vi "test FFT sound.vi"() -> ()   [LabVIEW 2013]
uses:
  <vilib>/measure/maspectr.llb/Power Spectrum and PSD Export Mode.ctl
  <vilib>/DAQmx/read.llb/DAQmx Read (Analog Wfm 1Chan NSamp).vi
  <vilib>/Analysis/2dsp.llb/Real FFT.vi
  <vilib>/Analysis/2dsp.llb/Power Spectrum (DBL).vi
  <vilib>/DAQmx/create/channels.llb/DAQmx Create Channel (AI-Voltage-Basic).vi
  <vilib>/DAQmx/configure/timing.llb/DAQmx Timing (Sample Clock).vi
  <vilib>/DAQmx/miscellaneous.llb/DAQmx Fill In Error Info.vi
  <vilib>/express/express analysis/Spectral/Block/exnSpectralBlock spectral measurements power poly.vi
  <vilib>/express/express analysis/Spectral/Block/exnSpectralBlock spectral measurements power WFM.vi
  <vilib>/measure/maspectr.llb/FFT Power Spectrum and PSD for 1 Chan.vi
  <vilib>/measure/maspectr.llb/FFT Spectrum (Mag-Phase) for 1 Chan.vi
  <vilib>/measure/maspectr.llb/FFT Spectrum (Real-Im) for 1 Chan.vi
  <vilib>/express/express analysis/Spectral/XNode/ExpressSpectralMeasurementsBlockNode.xnode
  <vilib>/Analysis/NI_AALPro.lvlib
  <vilib>/measure/NI_MAPro.lvlib
panel:
  out "Waveform Graph":cluster{"f0":dbl, "df":dbl, "magnitude":dbl[]}(graph)
  out "element":string
  in  "index (row)":i32
  in  "spectrum units table":string[][](table)=[["FFT", "N * V", "N/2 * Vpk"], ["Power Spectrum", "V^2", "1/2 * Vrms^2"], ["Auto Power Spectrum", "V^2", "Vrms^2"], ["Amplitude and Phase Spectrum", "V", "Vrms"], ["FFT Power Spectrum", "V^2", "Vrms^2"], ["FFT Power Spectral Density", "V^2/Hz", "Vrms^2/Hz"], ["FFT Spectrum (Mag-Phase)", "V", "Vrms"], ["FFT Spectrum (Real-Imag)", "V", "Vrms"]]
  in  "stop":bool
  out "phase spectrum":dbl[](array[numeric])
  out "spectral plot":cluster{"t":dbl, "t":dbl, "magnitude":dbl[]}(graph)={"t"=0.0, "t"=1.0, "magnitude"=[]}
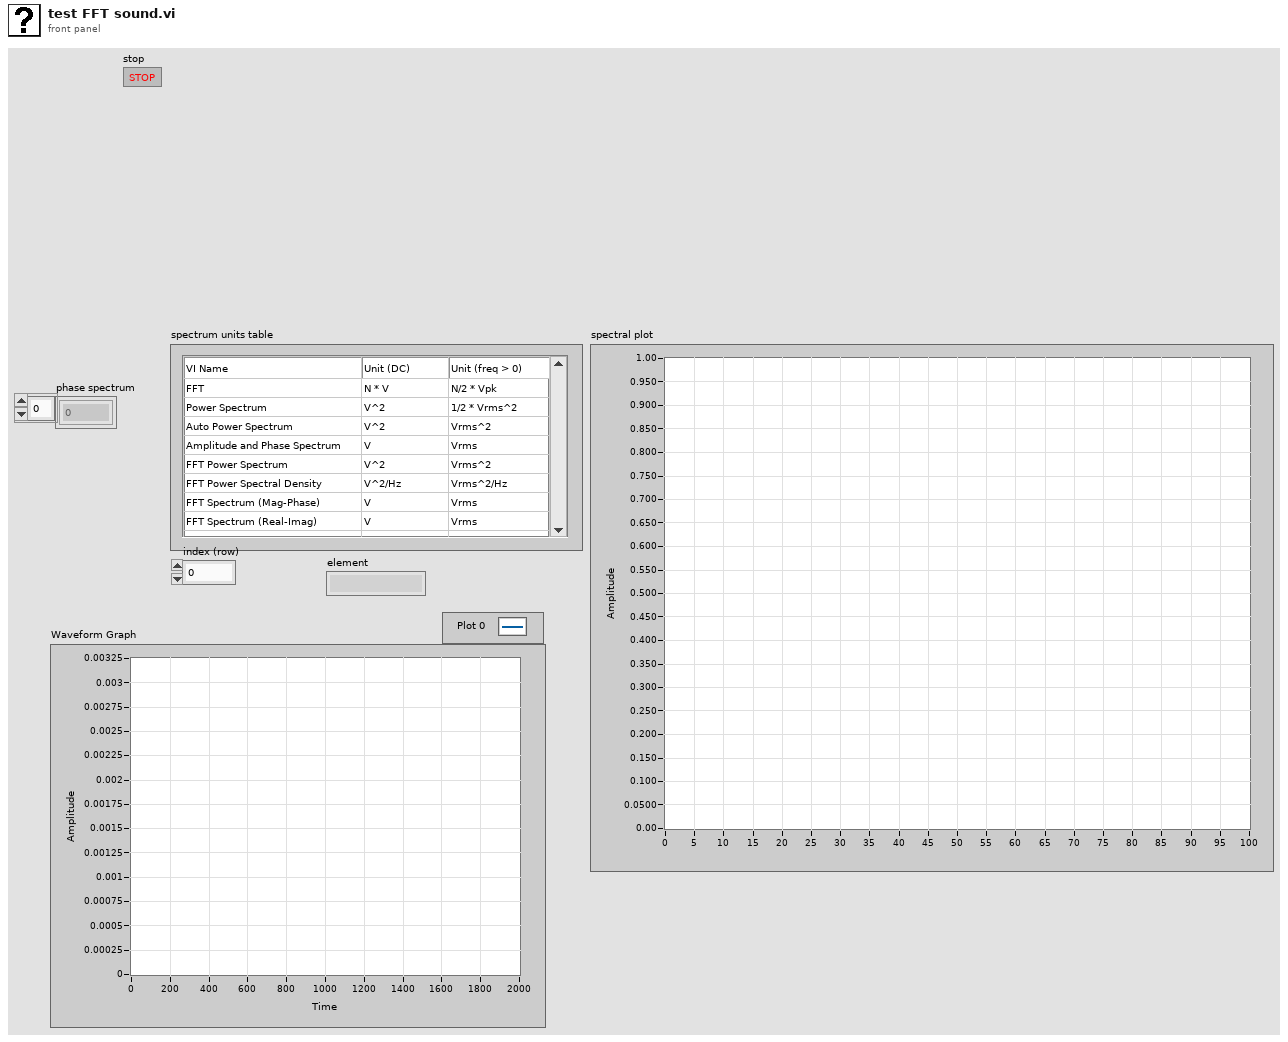
[diagram p1: front panel]
types:
  T1 = cluster{"averaging mode":u16, "weighting mode":u16, "number of averages":u32}
  T2 = cluster{"dB On (F)":bool, "unwrap phase (F)":bool, "convert to degree (F)":bool}
  T3 = enum16{"None ", "Hanning", "Hamming", "Blackman-Harris", "Exact Blackman", "Blackman", "Flat Top", "4 Term B-Harris ", "7 Term B-Harris", "Low Sidelobe"}
  T4 = typedef "NI_MAPro.lvlib/Power Spectrum and PSD Export Mode.ctl" = u16
  T5 = cluster{"f0":dbl, "df":dbl, "imaginary part":dbl[]}
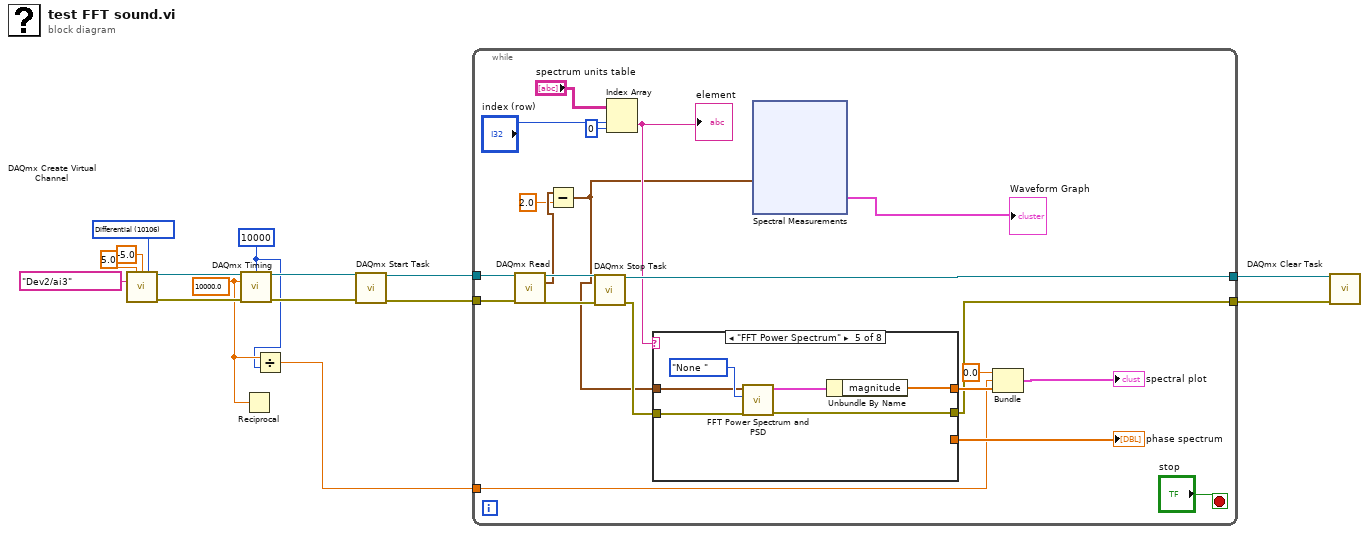
[diagram p0: block diagram]
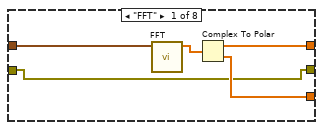
[diagram p2: hidden frame]
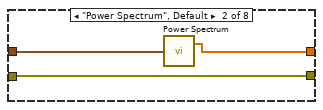
[diagram p3: hidden frame]
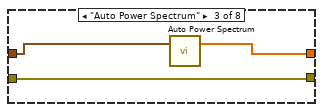
[diagram p4: hidden frame]
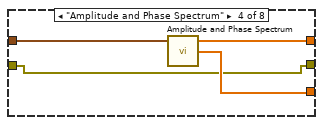
[diagram p5: hidden frame]
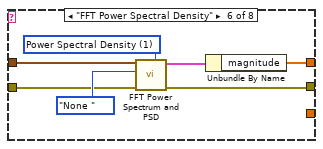
[diagram p6: hidden frame]
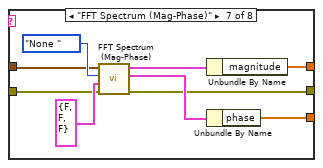
[diagram p7: hidden frame]
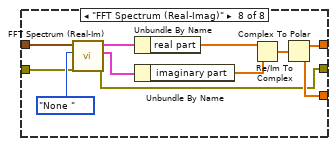
[diagram p8: hidden frame]
diagram:
  w3 = 10000.0 ("rate")
  w2 = 10000 ("samples per channel")
  w12 = 10106 items=["default"=-1, "RSE"=10083, "NRSE"=10078, "Differential"=10106, "Pseudodifferential"=12529] ("input terminal configuration")
  n1 = call-poly <vilib>:"DAQmx Create Virtual Channel.vi"("maximum value"=5.0, "minimum value"=-5.0, "input terminal configuration"=w12, "physical channels"=tag "Dev2/ai3") -> ("task out"=w11:refnum<k21>, "error out"=w10:errorcluster)  [unwired: 5 in, 5 out]
  n2 = call-poly <vilib>:"DAQmx Timing.vi"("task/channels in"=w11, "samples per channel"=w2, "rate"=w3, "error in"=w10) -> ("task out"=w9:refnum<k21>, "error out"=w8:errorcluster)  [unwired: 3 in, 7 out]
  n3 = Reciprocal(x=w3) -> ()  [unwired: 1 out]
  n4 = Divide(x=w3, y=w2) -> (x/y=w1:dbl)
  n5 = call <vilib>:"DAQmx Start Task.vi"("task/channels in"=w9, "error in"=w8) -> ("task out"=w6:refnum<k21>, "error out"=w7:errorcluster)  [unwired: 12 out]
  n6 = while {
    tunnel: w7 -> [w34]
    tunnel: w6 -> [w33]
    tunnel: [w32] -> w4
    tunnel: [w25] -> w5
    tunnel: w1 -> [w27]
    stop <- "stop" stop-if-true
    n7 = call-poly <vilib>:"DAQmx Read.vi"("task/channels in"=w33, "error in"=w34) -> ("task out"=w36:refnum<k21>, "data"=w17:waveform(dbl), "error out"=w35:errorcluster)  [unwired: 1 in, 10 out]
    n8 = Subtract(x=w17, y=2.0) -> (x-y=w18:waveform(dbl))
    n9 = call <vilib>:"DAQmx Stop Task.vi"("task/channels in"=w36, "error in"=w35) -> ("task out"=w32:refnum<k21>, "error out"=w26:errorcluster)  [unwired: 12 out]
    n10 = Index Array(array="spectrum units table", index (row)="index (row)", index (col)=0 ("disabled index (col)")) -> (element=w20:string)
    "element" <- w20
    n11 = case shown="\"FFT Power Spectrum\"" w20 {
      tunnel: [w49 w53 w56 w60 w65 w72 w81 w87] -> w30
      tunnel: [w48 _ _ w59 _ _ w78 w86] -> w28
      tunnel: [w46 w51 w54 w57 w63 w69 w76 w85] -> w25
      tunnel: w18 -> [w47 w52 w55 w58 w62 w68 w74 w84]
      tunnel: w26 -> [w46 w51 w54 w57 w61 w67 w75 w83]
      frame "FFT" {
        n12 = call-poly <vilib>:"FFT.vi"("X"=w47) -> ("FFT {X}"=w50:cdb[])  [unwired: 9 in, 1 out]
        n13 = Complex To Polar(r * e^(i*theta)=w50) -> (r=w49:dbl[], theta=w48:dbl[])
      }
      frame "Power Spectrum", Default {
        n14 = call-poly <vilib>:"Power Spectrum.vi"("X"=w52) -> ("Power Spectrum"=w53:dbl[])  [unwired: 1 out]
      }
      frame "Auto Power Spectrum" {
        n15 = call <vilib>:"Auto Power Spectrum.vi"("Signal (V)"=w55) -> ("Power Spectrum (V^2 rms)"=w56:dbl[])  [unwired: 1 in, 1 out]
      }
      frame "Amplitude and Phase Spectrum" {
        n16 = call <vilib>:"Amplitude and Phase Spectrum.vi"("Signal (V)"=w58) -> ("Amp Spectrum Phase (radians)"=w59:dbl[], "Amp Spectrum Mag (Vrms)"=w60:dbl[])  [unwired: 2 in, 1 out]
      }
      frame "FFT Power Spectrum" {
        n17 = call-poly <vilib>:"FFT Power Spectrum and PSD.vi"("error in (no error)"=w61, "window"=T3."None ", "time signal"=w62) -> ("error out"=w63:errorcluster, "Power Spectrum / PSD"=w66:cluster{"f0":dbl, "df":dbl, "magnitude":dbl[]})  [unwired: 5 in, 2 out]
        n18 = Unbundle By Name(w66) -> ("magnitude"=w65:dbl[])
      }
      frame "FFT Power Spectral Density" {
        w70 = T4 1 items=["Power Spectrum", "Power Spectral Density"] ("export mode")
        n19 = call-poly <vilib>:"FFT Power Spectrum and PSD.vi"("export mode"=w70, "error in (no error)"=w67, "window"=T3."None ", "time signal"=w68) -> ("error out"=w69:errorcluster, "Power Spectrum / PSD"=w73:cluster{"f0":dbl, "df":dbl, "magnitude":dbl[]})  [unwired: 4 in, 2 out]
        n20 = Unbundle By Name(w73) -> ("magnitude"=w72:dbl[])
      }
      frame "FFT Spectrum (Mag-Phase)" {
        n21 = call-poly <vilib>:"FFT Spectrum (Mag-Phase).vi"("error in (no error)"=w75, "view"=T2 {"dB On (F)"=FALSE, "unwrap phase (F)"=FALSE, "convert to degree (F)"=FALSE}, "window"=T3."None ", "time signal"=w74) -> ("error out"=w76:errorcluster, "phase"=w79:cluster{"f0":dbl, "df":dbl, "phase":dbl[]}, "magnitude"=w82:cluster{"f0":dbl, "df":dbl, "magnitude":dbl[]})  [unwired: 3 in, 2 out]
        n22 = Unbundle By Name(w82) -> ("magnitude"=w81:dbl[])
        n23 = Unbundle By Name(w79) -> ("phase"=w78:dbl[])
      }
      frame "FFT Spectrum (Real-Imag)" {
        n24 = call-poly <vilib>:"FFT Spectrum (Real-Im).vi"("error in (no error)"=w83, "window"=T3."None ", "time signal"=w84) -> ("error out"=w85:errorcluster, "imaginary part"=w91:T5, "real part"=w93:cluster{"f0":dbl, "df":dbl, "real part":dbl[]})  [unwired: 4 in, 2 out]
        n25 = Unbundle By Name(w93) -> ("real part"=w90:dbl[])
        n26 = Unbundle By Name(w91) -> ("imaginary part"=w89:dbl[])
        n27 = Re/Im To Complex(1:w89, 2:w90) -> (0:w88:cdb[])
        n28 = Complex To Polar(r * e^(i*theta)=w88) -> (r=w87:dbl[], theta=w86:dbl[])
      }
    }
    "phase spectrum" <- w28
    n29 = xnode "Spectral Measurements"("Signals"=w18) -> ("Power Spectrum"=→"Waveform Graph":cluster{"f0":dbl, "df":dbl, "magnitude":dbl[]})  [unwired: 1 in, 1 out]
    n30 = Bundle("t"=0.0, w27, "magnitude"=w30) -> (→"spectral plot":cluster{"t":dbl, dbl, "magnitude":dbl[]})  [unwired: 1 in]
  }
  n31 = call <vilib>:"DAQmx Clear Task.vi"("task in"=w4, "error in"=w5) -> ()  [unwired: 13 in, 1 out]
